vi "finishup.vi"(8 "error in (no error)":errorcluster, 11 "FringeTestingViewer in":refnum<class "FringeTestingViewer.lvclass">) -> (0 "error out":errorcluster, 3 "FringeTestingViewer out":refnum<class "FringeTestingViewer.lvclass">)   [LabVIEW 2009, in "Views.lvlib" / "Camera.lvlib" / "FringeTestingViewer.lvclass"]
uses:
  FringeTestingViewer.lvclass
  FringeTestingViewer.lvclass/FringeTestingViewer.ctl
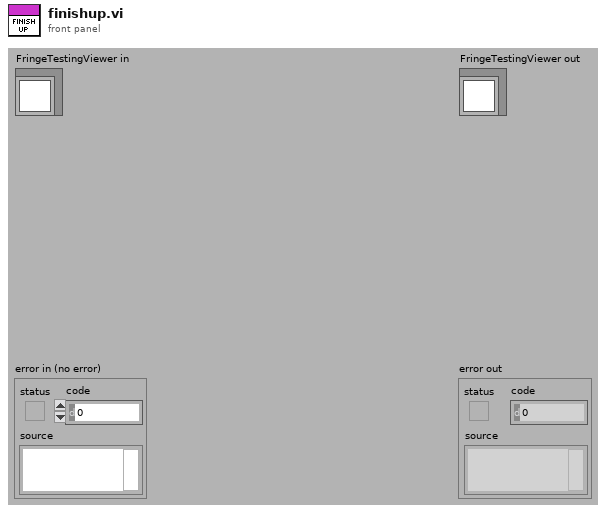
[diagram p1: front panel]
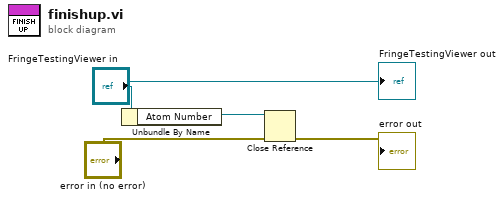
[diagram p0: block diagram]
diagram:
  n1 = Unbundle By Name("FringeTestingViewer in") -> ("Atom Number"=w4:refnum<vi>)
  n2 = Close Reference(reference=w4, error in (no error)="error in (no error)") -> (error out=→"error out":errorcluster)
  "FringeTestingViewer out" <- "FringeTestingViewer in"
